vi "SGA.vi"(0 "System no.":i32=1 min=1 max=4 step=1, 1 "Board":i32=1 min=1 max=5 step=1, 3 "Gain":i32=10 min=0 max=1000 step=10, 5 "error in":errorcluster) -> (14 "Controller error":bool, 19 "error out":errorcluster)   [LabVIEW 2020]
doc: "Sets the gain value for the optical input. See system manual for allowable gain values. Controller error is TRUE if selected system reports an error code which is not 0."
uses:
  Syntax.ctl
  Global1.vi
panel:
  # "Sets the gain value for the optical input. See system\nmanual for allowable gain values."
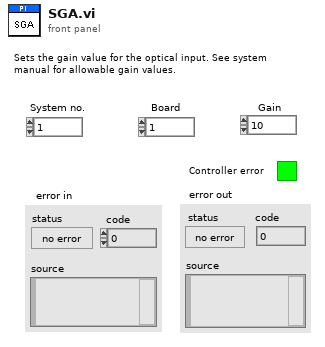
[diagram p1: front panel]
types:
  T1 = typedef "Syntax.ctl" = enum16{"GCS 1.0", "GCS 2.0", "GCS 3.0"}
  T2 = enum16{"Disable error check", "Force error check", "Use global settings"}
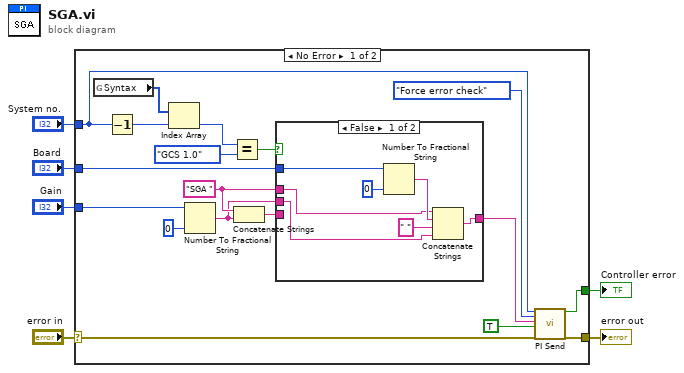
[diagram p0: block diagram]
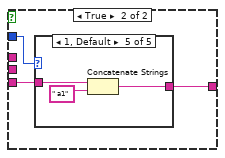
[diagram p2: hidden frame]
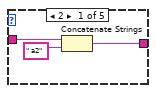
[diagram p3: hidden frame]
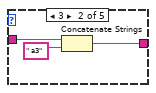
[diagram p4: hidden frame]
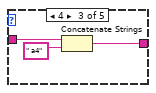
[diagram p5: hidden frame]
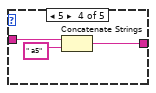
[diagram p6: hidden frame]
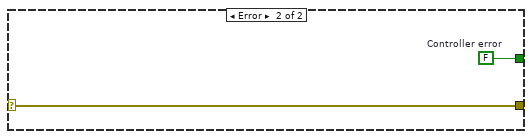
[diagram p7: hidden frame]
diagram:
  n1 = case shown="No Error" "error in" {
    selector: "error in" -> [w11 w51]
    tunnel: [w10 w51] -> w6
    tunnel: [w9 w50] -> w5
    tunnel: "Gain" -> [w24 _]
    tunnel: "Board" -> [w21 _]
    tunnel: "System no." -> [w14 _]
    frame No Error {
      w13 = "SGA "
      n2 = global read "Global1.vi" "Syntax"() -> (w18:T1[])
      n3 = Decrement(x=w14) -> (x-1=w17:i32)
      n4 = Index Array(array=w18, index=w17) -> (element=w16:T1)
      n5 = Number To Fractional String(number=w24, precision (6)=i16 0) -> (F-format string=w12:string)  [unwired: 2 out]
      n6 = Equal?(x=w16, y=Syntax."GCS 1.0") -> (x = y?=w15:bool)
      n7 = Concatenate Strings(w13, w12) -> (w19:string)
      n8 = case shown="False" w15 {
        tunnel: w21 -> [w27 w34]
        tunnel: [w25 w33] -> w20
        tunnel: w19 -> [_ w32]
        tunnel: w13 -> [w28 _]
        tunnel: w12 -> [w26 _]
        frame False {
          n9 = Number To Fractional String(number=w27, precision (6)=i16 0) -> (F-format string=w30:string)  [unwired: 2 out]
          n10 = Concatenate Strings(w28, w30, " ", w26) -> (w25:string)
        }
        frame True {
          n11 = case shown="1, Default" w34 {
            tunnel: w32 -> [w37 w40 w43 w46 w49]
            tunnel: [w35 w38 w41 w44 w47] -> w33
            frame 2 {
              n12 = Concatenate Strings(w37, " a2" ("Substring")) -> (w35:string)
            }
            frame 3 {
              n13 = Concatenate Strings(w40, " a3" ("Substring")) -> (w38:string)
            }
            frame 4 {
              n14 = Concatenate Strings(w43, " a4" ("Substring")) -> (w41:string)
            }
            frame 5 {
              n15 = Concatenate Strings(w46, " a5" ("Substring")) -> (w44:string)
            }
            frame 1, Default {
              n16 = Concatenate Strings(w49, " a1" ("Substring")) -> (w47:string)
            }
          }
        }
      }
      n17 = call "PI Send.vi"("System no."=w14, "Error check settings"=T2."Force error check", "String to send"=w20, "Attach termination char.?"=TRUE ("Attach Linefeed?"), "error in"=w11) -> ("Controller error"=w9:bool, "error out"=w10:errorcluster)  [unwired: 1 in, 12 out]
    }
    frame Error {
      w50 = FALSE  # Controller error
    }
  }
  "error out" <- w6
  "Controller error" <- w5
